vi "Match.vi"(8 "error in (no error)":errorcluster, 10 "Token Type":i32, 11 "Alpaca Parser in":refnum<class "Parser.lvclass">) -> (0 "error out":errorcluster, 3 "Alpaca Parser out":refnum<class "Parser.lvclass">)   [LabVIEW 2019, in "JKI JSON Serialization.lvlib" / "Parser.lvclass"]
doc: "JKI JSON 1.1.10.37\nTomi Maila - JKI\nCopyright (c) 2017, JKI"
uses:
  Parser.lvclass
  Parser.lvclass/Parser.ctl
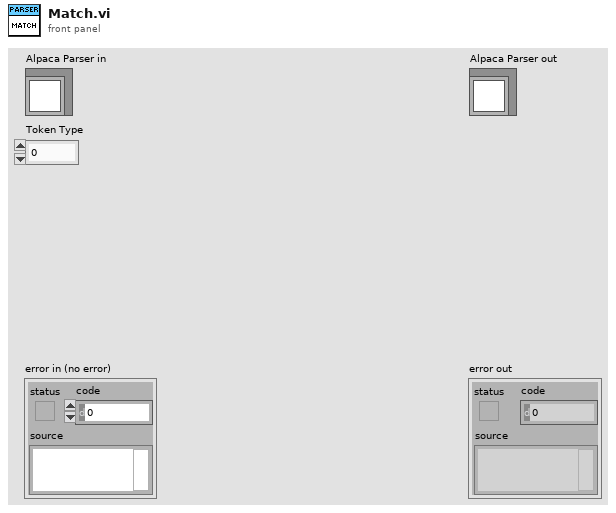
[diagram p1: front panel]
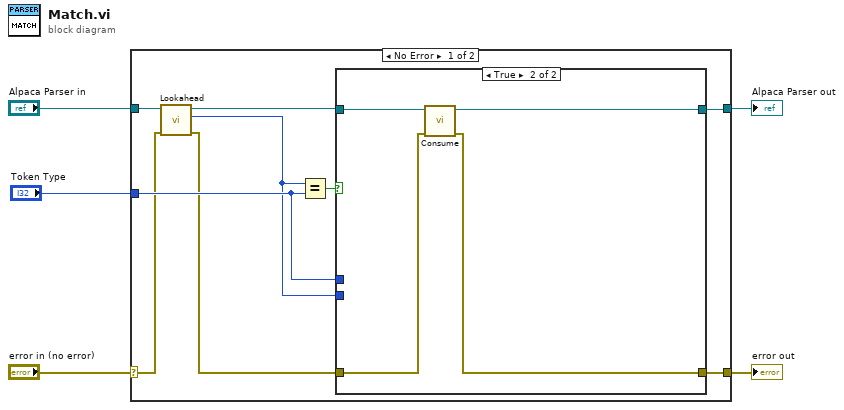
[diagram p0: block diagram]
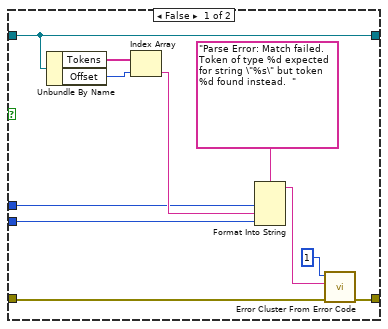
[diagram p2: hidden frame]
diagram:
  n1 = case shown="No Error" "error in (no error)" {
    selector: "error in (no error)" -> [w8 w31]
    tunnel: [w13 w31] -> w4
    tunnel: [w14 w30] -> w2
    tunnel: "Alpaca Parser in" -> [w10 w30]
    tunnel: "Token Type" -> [w11 _]
    frame No Error {
      n2 = call "Lookahead.vi"("error in (no error)"=w8, "Alpaca Parser in"=w10) -> ("error out"=w7:errorcluster, "Lookahead Type"=w6:i32, "Alpaca Parser out"=w9:refnum<class "Parser.lvclass">)  [unwired: 6 in, 1 out]
      n3 = Equal?(x=w6, y=w11) -> (x = y?=w12:bool)
      n4 = case shown="True" w12 {
        tunnel: w9 -> [w20 w29]
        tunnel: [w20 w28] -> w14
        tunnel: [w25 w27] -> w13
        tunnel: w7 -> [w24 w26]
        tunnel: w6 -> [w15 _]
        tunnel: w11 -> [w16 _]
        frame False {
          n5 = Unbundle By Name(w20) -> ("Tokens"=w19:string[], "Offset"=w18:i32)
          n6 = Index Array(array=w19, index=w18) -> (element=w17:string)
          n7 = Format Into String(format string="Parse Error: Match failed. Token of type %d expected for string \"%s\" but token %d found instead.  " ("error message (\"\")"), w16, w17, w15) -> (resulting string=w21:string)  [unwired: 2 in, 1 out]
          n8 = call <vilib>:"Error Cluster From Error Code.vi"("error in (no error)"=w24, "error message (\"\")"=w21, "error code (0)"=1) -> ("error out"=w25:errorcluster)  [unwired: 6 in]
        }
        frame True {
          n9 = call-dynamic "Consume.vi"("error in (no error)"=w26, "Alpaca Parser in"=w29) -> ("error out"=w27:errorcluster, "Alpaca Parser out"=w28:refnum<class "Parser.lvclass">)  [unwired: 8 in]
        }
      }
    }
    frame Error {
    }
  }
  "error out" <- w4
  "Alpaca Parser out" <- w2
